vi "klinger ErrorHandler.vi"(2 "error in (no error)":errorcluster, 3 "Message D'erreur":string) -> (0 "error out":errorcluster, 1 "Erreur":bool)   [LabVIEW 2010]
doc: "Ce VI vérifie si une erreur a eu lieu et si c'est le cas, il affiche un message. Si l'erreur provient du contrôleur, celle-ci est ensuite effacée."
uses:
  <vilib>/Utility/error.llb/DialogType.ctl
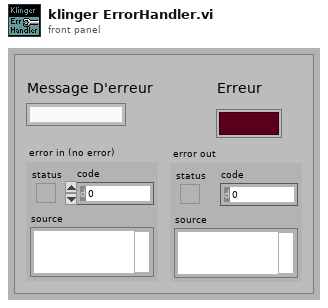
[diagram p1: front panel]
types:
  T1 = typedef "DialogType.ctl" = u16
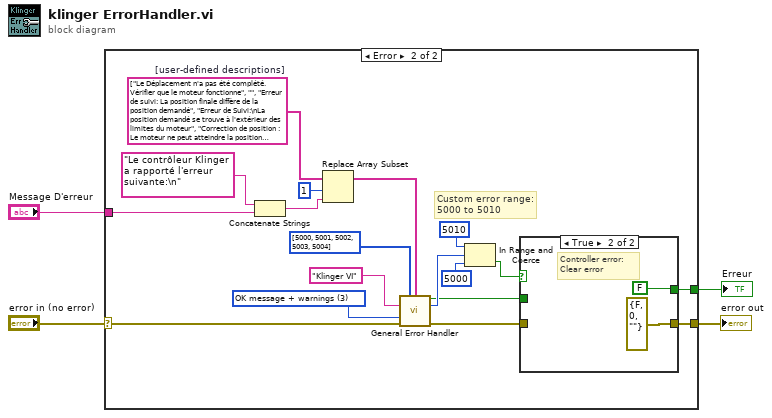
[diagram p0: block diagram]
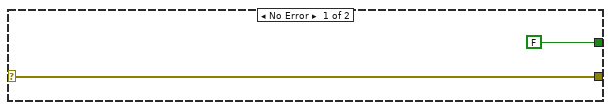
[diagram p2: hidden frame]
diagram:
  n1 = case shown="Error" "error in (no error)" {
    selector: "error in (no error)" -> [w6 w15]
    tunnel: [w6 w13] -> w4
    tunnel: [FALSE ("error?") w8] -> w3
    tunnel: "Message D'erreur" -> [_ w16]
    frame No Error {
    }
    frame Error {
      w17 = string[] ["Le Déplacement n'a pas été complété. Vérifier que le moteur fonctionne", "", "Erreur de suivi: La position finale diffère de la position demandé", "Erreur de Suivi:\nLa position demandé se trouve à l'extérieur des limites du moteur", "Correction de position : Le moteur ne peut atteindre la position demandée"]  # [user-defined descriptions]
      w24 = T1 3 items=["no dialog", "OK message", "continue or stop message", "OK message + warnings", "continue/stop + warnings"] ("type of dialog (OK msg:1)")
      # "Custom error range:\n5000 to 5010"
      n2 = Concatenate Strings("Le contrôleur Klinger a rapporté l'erreur suivante:\n" ("string"), w16) -> (w19:string)
      n3 = Replace Array Subset(array=w17, new element=w19, index=1) -> (w20:string[])
      n4 = call <vilib>:"General Error Handler.vi"("[user-defined codes]"=i32[] [5000, 5001, 5002, 5003, 5004], "[user-defined descriptions]"=w20, "[error source] (\" \")"="Klinger VI" ("[error source] (\" \")"), "type of dialog (OK msg:1)"=w24, "error in (no error)"=w15) -> ("error?"=w7:bool, "code out"=w12:i32, "error out"=w14:errorcluster)  [unwired: 6 in, 2 out]
      n5 = In Range and Coerce(upper limit=5010, x=w12, lower limit=5000) -> (In Range?=w9:bool)  [unwired: 1 out]
      n6 = case shown="True" w9 {
        tunnel: [w26 errorcluster {"status"=FALSE, "code"=0, "source"=""} ("error out")] -> w13
        tunnel: w14 -> [w26 _]
        tunnel: [w25 FALSE ("error?")] -> w8
        tunnel: w7 -> [w25 _]
        frame False {
          # "Not a controller error:\nPass error out"
        }
        frame True {
          # "Controller error:\nClear error"
        }
      }
    }
  }
  "Erreur" <- w3
  "error out" <- w4
